vi "fgv_PwrPak7_config.vi"(7 "cmd":enum16{"read", "write"}(ring), 8 "error in":errorcluster, 11 "PP7 cfg":T2={"PwrPak7 Port"="COM5", "heading select"=enum."NARROW_INT", "mode select"=[enum."INS_RTKFIXED", enum."NARROW_FLOAT"], "ref_center"={"x"=38.0, "y"=127.0}}) -> (0 "error out":errorcluster, 3 "PP7 cfg out":T2={"PwrPak7 Port"="COM5", "heading select"=enum."NARROW_INT", "mode select"=[enum."INS_RTKFIXED", enum."NARROW_FLOAT"], "ref_center"={"x"=38.0, "y"=127.0}})   [LabVIEW 2019]
uses:
  Ctrl/gnss_heading-key.ctl
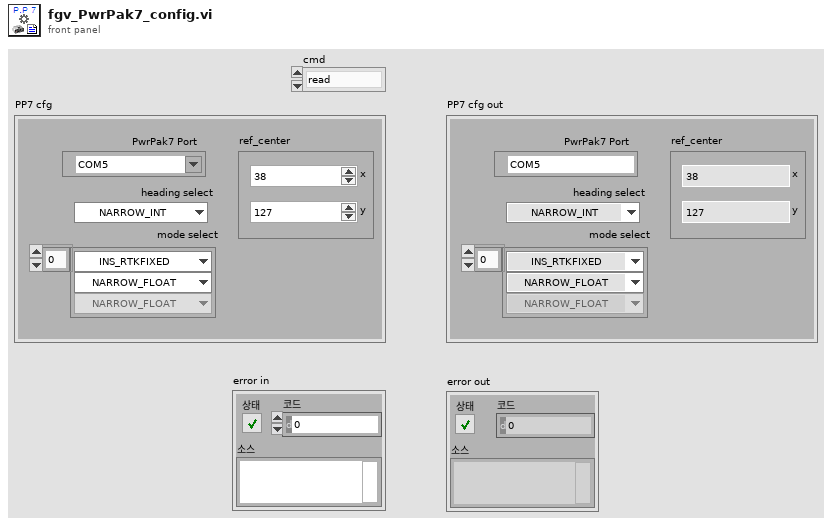
[diagram p1: front panel]
types:
  T1 = typedef "gnss_heading-key.ctl" = enum16{"NARROW_FLOAT", "NARROW_INT", "RTK_DIRECT_INS", "INS_SBAS", "INS_PSRSP", "INS_RTKFLOAT", "INS_RTKFIXED"}
  T2 = cluster{"PwrPak7 Port":refnum<visa-resource-name>, "heading select":T1, "mode select":T1[], "ref_center":cluster{"x":dbl, "y":dbl}}
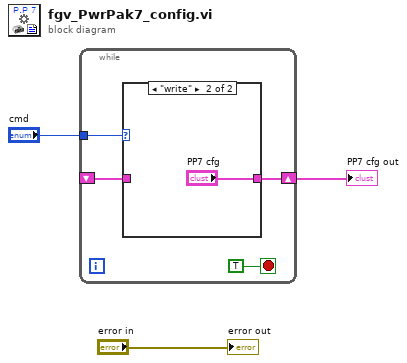
[diagram p0: block diagram]
diagram:
  n1 = while {
    tunnel: "cmd" -> [w6]
    shift-right: [w5] -> w1
    shift-left: _ -> [w4]
    stop <- TRUE stop-if-true
    n2 = case shown="\"write\"" w6 {
      tunnel: [w8 "PP7 cfg"] -> w5
      tunnel: w4 -> [w8 _]
      frame "read", Default {
      }
      frame "write" {
      }
    }
  }
  "PP7 cfg out" <- w1
  "error out" <- "error in"
